vi "save and clear data.vi"(8 "error in (no error)":errorcluster, 11 "Data Log in":refnum<class "Data Log.lvclass">) -> (0 "error out":errorcluster, 3 "Data Log out":refnum<class "Data Log.lvclass">)   [LabVIEW 2025, in "Data Log.lvclass"]
uses:
  Data Log.lvclass
  Data Log.lvclass/Data Log.ctl
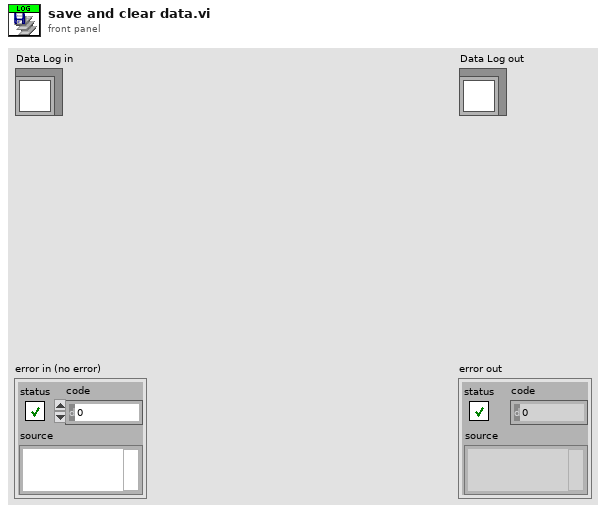
[diagram p1: front panel]
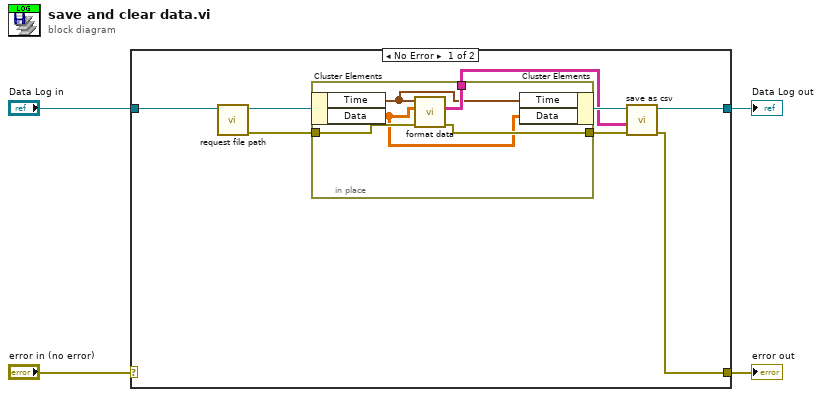
[diagram p0: block diagram]
diagram:
  n1 = case shown="No Error" "error in (no error)" {
    selector: "error in (no error)" -> [_ w19]
    tunnel: [w5 w19] -> w3
    tunnel: [w11 w18] -> w1
    tunnel: "Data Log in" -> [w10 w18]
    frame No Error {
      n2 = call-dynamic "request file path.vi"("Data Log in"=w10) -> ("error out"=w8:errorcluster, "Data Log out"=w9:refnum<class "Data Log.lvclass">)  [unwired: 8 in, 1 out]
      n3 = in-place {
        in-place-border: w8 -> [w17]
        in-place-border: [w16] -> w7
        in-place-border: [w15] -> w6
        n4 = in-place-cluster #1(w9) -> ("Time"=w14:timestamp[], "Data"=w13:dbl[][])
        n5 = call "format data.vi"("error in (no error)"=w17, "Data Array"=w13, "Date/Time Array"=w14) -> ("error out"=w16:errorcluster, "Data"=w15:string[][])  [unwired: 7 in]
        n6 = in-place-cluster #1("Time"=w14, "Data"=w13) -> (w12:refnum<class "Data Log.lvclass">)
      }
      n7 = call-dynamic "save as csv.vi"("error in (no error)"=w7, "Data"=w6, "Data Log in"=w12) -> ("error out"=w5:errorcluster, "Data Log out"=w11:refnum<class "Data Log.lvclass">)  [unwired: 7 in]
    }
    frame Error {
    }
  }
  "error out" <- w3
  "Data Log out" <- w1
